vi "Months_Total_Pay.vi"() -> ()   [LabVIEW 2022 SP3]
panel:
  out "?":dbl format="$ %#_10f"
  # "Months_Total_Pay:\nAssume you begin getting $0.01 a day. and each day this pay doubles.\nAfter 30 days, you would have earned a total of"
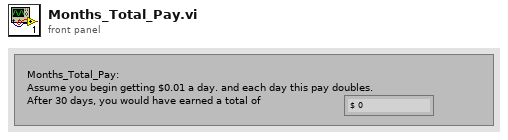
[diagram p1: front panel]
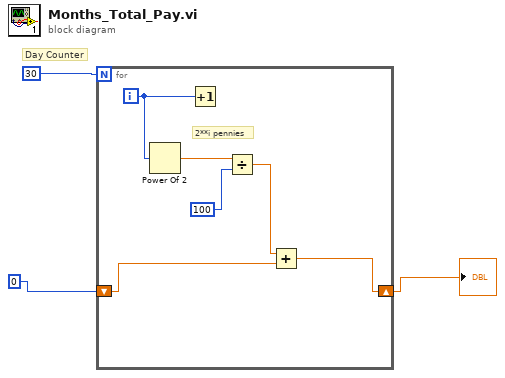
[diagram p0: block diagram]
diagram:
  # "Day Counter"
  n1 = for {
    N: 30 -> [_]
    shift-right: [w5] -> w2
    shift-left: 0 -> [w4]
    i -> [w9]
    # "2**i pennies"
    n2 = Power Of 2(x=w9) -> (2^x=w7:dbl)
    n3 = Increment(x=w9) -> ()  [unwired: 1 out]
    n4 = Divide(x=w7, y=100) -> (x/y=w6:dbl)
    n5 = Add(x=w6, y=w4) -> (x+y=w5:dbl)
  }
  "?" <- w2
